vi "Analyze.vi"(8 "error in (no error)":errorcluster, 10 "Image in":T1, 11 "Analyze Distanz in":refnum<class "Analyze Distanz.lvclass">) -> (0 "error out":errorcluster, 1 "Result":refnum<class "Analyze Results Base.lvclass">, 2 "Image out":T1, 3 "Analyze Distanz out":refnum<class "Analyze Distanz.lvclass">)   [LabVIEW 2020, in "Analyze.lvlib" / "Analyze Distanz.lvclass"]
uses:
  Analyze Distanz.lvclass
  C:/POLARIS Programme/POLARIS-AS-3-Cams/Submodules/HIJ Vision/Analyze/Analyze Classes/Analyze BaseClass/Analyze BaseClass/Analyze BaseClass.lvclass
  <vilib>/vision/Image Controls.llb/IMAQ Image.ctl
  Results and Overlays/Results Base/Analyze Results Base.lvclass
  Results and Overlays/Results Distance/Analyze Results Distanz.lvclass
  C:/POLARIS Programme/POLARIS-AS-3-Cams/Submodules/HIJ Vision/Analyze/Results and Overlays/Results Base/Analyze Results Base.lvclass
  Results and Overlays/Results Distance/Analyze Results Distanz.lvclass/Analyze Results Distanz.ctl
  Results and Overlays/Results Distance/Write Distances.vi
  Results and Overlays/Results Distance/Write Overlay Positions.vi
  Analyze BaseClass/Analyze BaseClass/Analyze BaseClass.lvclass
  Utility/POLARIS Vision utility.lvlib
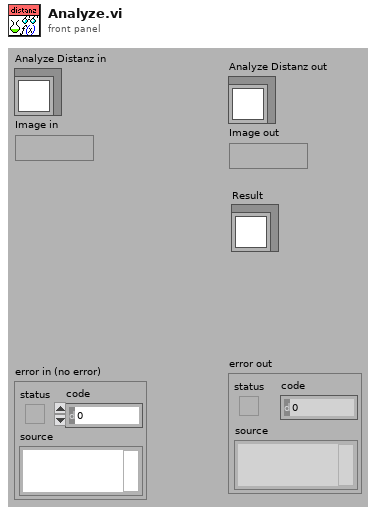
[diagram p1: front panel]
types:
  T1 = typedef "IMAQ Image.ctl" = refnum<image>
  T2 = typedef "ROI Descriptor" = cluster{"Global Rectangle":i32[], "Contours":cluster{"ID":enum32{"External", "Internal"}, "Type":u32, "Coordinates":i32[]}[]}
  T3 = cluster{"ID":enum32{"External", "Internal"}, "Type":u32, "Coordinates":i32[]}[]
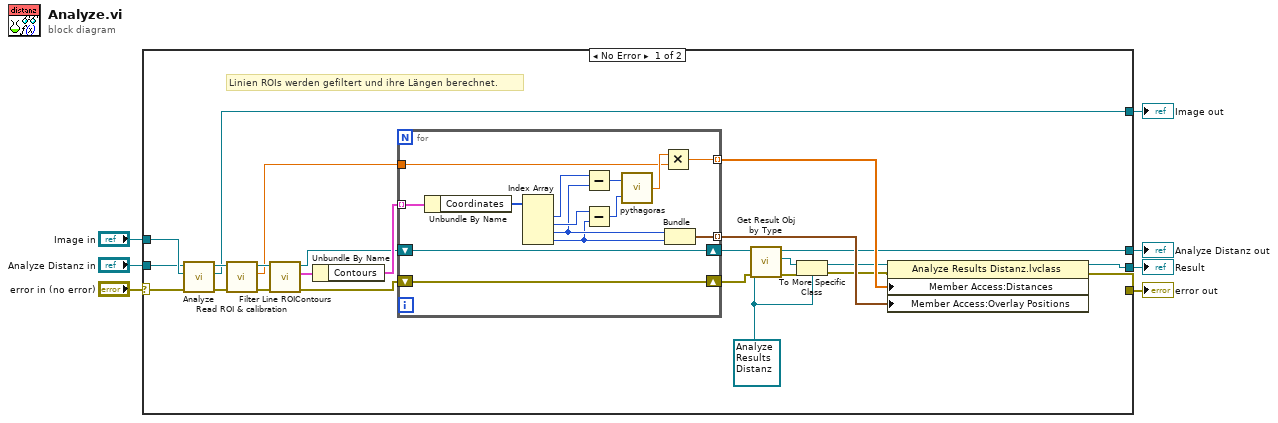
[diagram p0: block diagram]
diagram:
  n1 = case shown="No Error" "error in (no error)" {
    selector: "error in (no error)" -> [w8 w49]
    tunnel: "Image in" -> [w25 w47]
    tunnel: [w22 w47] -> w6
    tunnel: [w19 _] -> w5
    tunnel: "Analyze Distanz in" -> [w17 w48]
    tunnel: [w16 w48] -> w3
    tunnel: [w9 w49] -> w2
    frame No Error {
      w12 = refnum<class "Analyze Results Distanz.lvclass"> refnum ("Analyze Results Distanz.lvclass")
      # "Linien ROIs werden gefiltert und ihre Längen berechnet."
      n2 = call-parent "Analyze.vi"("error in (no error)"=w8, "Image in"=w25, "Analyze BaseClass in"=w17) -> ("error out"=w23:errorcluster, "Image out"=w22:T1, "Analyze BaseClass out"=w24:refnum<class "Analyze Distanz.lvclass">)  [unwired: 5 in, 1 out]
      n3 = call-dynamic "Read ROI & calibration.vi"("error in (no error)"=w23, "Analyze BaseClass in"=w24) -> ("error out"=w32:errorcluster, "calibration mm/px"=w28:dbl[unit], "Analyze BaseClass out"=w31:refnum<class "Analyze Distanz.lvclass">)  [unwired: 6 in, 1 out]
      n4 = call-dynamic "Filter Line ROIContours.vi"("error in (no error)"=w32, "Analyze BaseClass in"=w31) -> ("error out"=w26:errorcluster, "Line contours"=w30:T2, "Analyze BaseClass out"=w27:refnum<class "Analyze Distanz.lvclass">)  [unwired: 7 in]
      n5 = Unbundle By Name(w30) -> ("Contours"=w29:T3)
      n6 = for {
        tunnel: w29 -> [w46] mode=indexing
        tunnel: w28 -> [w39]
        shift-right: [w38] -> w18
        shift-left: w27 -> [w38]
        shift-right: [w37] -> w13
        shift-left: w26 -> [w37]
        tunnel: [w33] -> w21 mode=indexing
        tunnel: [w34] -> w20 mode=indexing
        n7 = Unbundle By Name(w46) -> ("Coordinates"=w45:i32[])
        n8 = Index Array(array=w45) -> (element #1=w43:i32, element #2=w42:i32, element #3=w36:i32, element #4=w35:i32)  [unwired: 4 in]
        n9 = Subtract(x=w43, y=w36) -> (x-y=w44:i32)
        n10 = Subtract(x=w42, y=w35) -> (x-y=w41:i32)
        n11 = call "pythagoras.vi"("b"=w41, "a"=w44) -> ("c"=w40:dbl)
        n12 = Multiply(x=w40, y=w39) -> (x*y=w33:dbl[unit])
        n13 = Bundle(w36, w35) -> (w34:cluster{i32, i32})  [unwired: 1 in]
      }
      n14 = call "Get Result Obj by Type.vi"("error in (no error)"=w13, "Parameter Type"=w12, "Analyze BaseClass in"=w18) -> ("error out"=w15:errorcluster, "Parameter"=w14:refnum<class "Analyze Results Base.lvclass">, "Analyze BaseClass out"=w16:refnum<class "Analyze Distanz.lvclass">)  [unwired: 5 in, 1 out]
      n15 = To More Specific Class(target class=w12, reference=w14, error in=w15) -> (specific class reference=w11:refnum<class "Analyze Results Distanz.lvclass">, error out=w10:errorcluster)
      n16 = property class="Analyze Results Distanz.lvclass"(reference=w11, error in=w10, "Member Access:Distances"=w21, "Member Access:Overlay Positions"=w20) -> (reference out=w19:refnum<class "Analyze Results Distanz.lvclass">, error out=w9:errorcluster)
    }
    frame Error {
    }
  }
  "error out" <- w2
  "Analyze Distanz out" <- w3
  "Image out" <- w6
  "Result" <- w5
